vi "Create 5792 Half Rate.vi"() -> (4 "sync.resources":T1)   [LabVIEW 2013, in "ni579x Synchronization v1 FPGA.lvlib"]
doc: "Create and initialize the resources for the Synchronization library appropriate for the NI 5792 FAM (synchronizing to the half rate clock).\n\n<B>Output Parameters</B>\n\n<B>sync.resources</B> is a new Synchronization instance."
uses:
  <instrlib>/ni579x/Synchronization/v1/FPGA/ni579x Synchronization v1 FPGA.lvlib
  <instrlib>/ni579x/Synchronization/v1/FPGA/Implementation/Resources.ctl
  <vilib>/rvi/eio/common/nirviEmuReportErrorAndStop.vi
  <vilib>/rvi/DataTransferAndStorage/Container/Common/niFpgaContainerSetEmuInfo.vi
  <vilib>/rvi/DataTransferAndStorage/Container/Common/niFpgaContainerGetUniqueNameForEmu.vi
  <vilib>/rvi/LocalResourceManager/LocalResourceManager.xnode
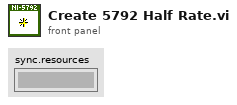
[diagram p1: front panel]
types:
  T1 = typedef "ni579x Synchronization v1 FPGA.lvlib/Resources.ctl" = cluster{"master":refnum<k21>, "meas.enable":refnum<k21>, "meas.ready":refnum<k21>, "meas.arm":refnum<k21>, "meas.valid":refnum<k21>, "meas.value":refnum<k21>, "meas.oversample clock":refnum<k21>, "meas.oversample factor":refnum<k21>, "cptr":refnum<k21>, "cptr.adjust":refnum<k21>, "cptr.period":refnum<k21>}
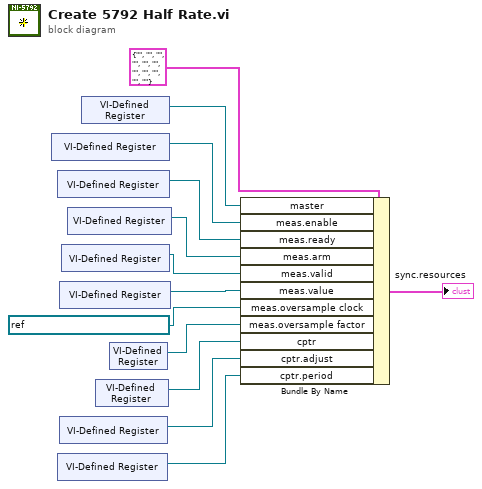
[diagram p0: block diagram]
diagram:
  n1 = xnode "VI-Defined Register"() -> ("Register Out"=w12:refnum<k21>)
  n2 = xnode "VI-Defined Register"() -> ("Register Out"=w13:refnum<k21>)
  n3 = xnode "VI-Defined Register"() -> ("Register Out"=w8:refnum<k21>)
  n4 = xnode "VI-Defined Register"() -> ("Register Out"=w6:refnum<k21>)
  n5 = xnode "VI-Defined Register"() -> ("Register Out"=w7:refnum<k21>)
  n6 = xnode "VI-Defined Register"() -> ("Register Out"=w5:refnum<k21>)
  n7 = xnode "VI-Defined Register"() -> ("Register Out"=w4:refnum<k21>)
  n8 = xnode "VI-Defined Register"() -> ("Register Out"=w9:refnum<k21>)
  n9 = xnode "VI-Defined Register"() -> ("Register Out"=w3:refnum<k21>)
  n10 = xnode "VI-Defined Register"() -> ("Register Out"=w1:refnum<k21>)
  n11 = Bundle By Name(cluster=T1 {"master"="", "meas.enable"="", "meas.ready"="", "meas.arm"="", "meas.valid"="", "meas.value"="", "meas.oversample clock"="", "meas.oversample factor"="", "cptr"="", "cptr.adjust"="", "cptr.period"=""} ("sync.resources"), "master"=w9, "meas.enable"=w12, "meas.ready"=w13, "meas.arm"=w4, "meas.valid"=w5, "meas.value"=w6, "meas.oversample clock"=refnum<k21> "IO Module\\Sample Clock" ("sync.meas.FPGA Oversample Clock"), "meas.oversample factor"=w1, "cptr"=w3, "cptr.adjust"=w7, "cptr.period"=w8) -> (→"sync.resources":T1)
